vi "Open.vi"   [LabVIEW 2011, in "LVH-Xbox-One-Controller.lvlib"]
uses:
  LVH-Xbox-One-Controller.lvlib
  Test Apps/Async Worker.vi
types:
  T1 = cluster{"A":refnum<user-event>, "B":refnum<user-event>}
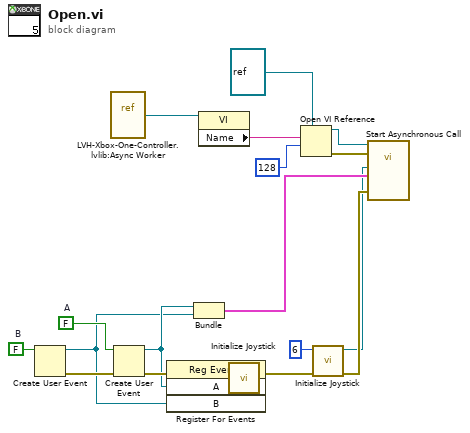
[diagram p0: block diagram]
diagram:
  w16 = FALSE  # B
  w17 = FALSE  # A
  n1 = Create User Event(user event datatype=w16) -> (user event=w11:refnum<user-event>, error out=w15:errorcluster)  [unwired: 1 in]
  n2 = vi-ref "LVH-Xbox-One-Controller.lvlib:Async Worker.vi"() -> (w9:refnum<vi>)
  n3 = Create User Event(user event datatype=w17, error in=w15) -> (user event=w12:refnum<user-event>, error out=w14:errorcluster)
  n4 = register-events(error in=w14, w12, w11) -> (error out=w10:errorcluster)  [unwired: 1 in, 1 out]
  n5 = Bundle("A"=w12, "B"=w11) -> (w2:T1)  [unwired: 1 in]
  n6 = property class="VI"(reference=w9) -> ("Name"=w4:string)  [unwired: 1 in, 2 out]
  n7 = call <vilib>:"Initialize Joystick.vi"() -> ()  [unwired: 10 in, 2 out]
  n8 = Open VI Reference(type specifier VI Refnum (for type only)=refnum<vi> refnum, vi path=w4, options=128) -> (vi reference=w6:refnum<vi>, error out=w5:errorcluster)  [unwired: 3 in]
  n9 = call <vilib>:"Initialize Joystick.vi"("error in (no error)"=w10, "device index"=6) -> ("error out"=w3:errorcluster, "device ID"=w1:refnum<k1>)  [unwired: 8 in]
  n10 = call-by-ref "Start Asynchronous Call"(reference=w6, error in=w5, 8:"error in (no error)"=w3, "Events"=w2, "Controller Ref"=w1) -> ()  [unwired: 6 in, 5 out]
